vi "FitsOpenFile.vi"(8 "error in (no error)":errorcluster, 10 "filename":string, 11 "CFitsIO in":refnum<class "CFitsIO.lvclass">) -> (0 "error out":errorcluster, 1 "result":i32, 2 "fp out":u64, 3 "CFitsIO out":refnum<class "CFitsIO.lvclass">)   [LabVIEW 2016, in "CFitsIO.lvclass"]
uses:
  CFitsIO.lvclass
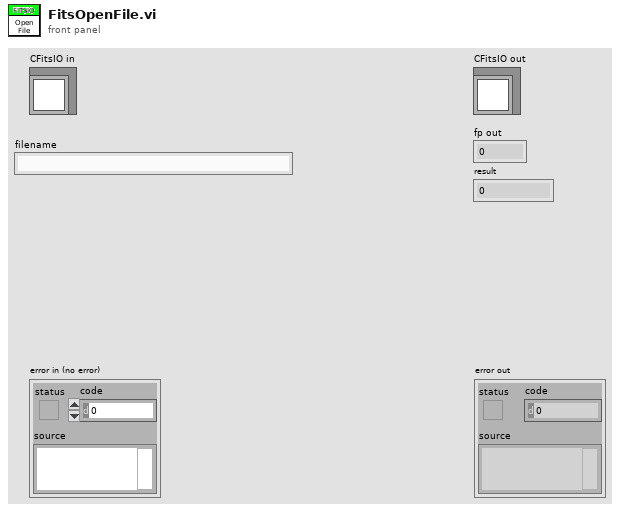
[diagram p1: front panel]
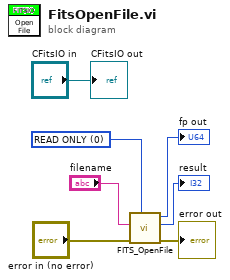
[diagram p0: block diagram]
diagram:
  w3 = 0 items=["READ ONLY", "READ/WRITE"] ("mode")
  n1 = call "FITS_OpenFile.vi"("mode"=w3, "error in"="error in (no error)", "filename"="filename") -> ("error out"=→"error out":errorcluster, "result"=→"result":i32, "fp out"=→"fp out":u64)  [unwired: 6 in]
  "CFitsIO out" <- "CFitsIO in"
